vi "Get Step Index from Tree Tag.vi"(11 "Tree Tag":string) -> (2 "Step Param String":string, 3 "Step Index":i32)   [LabVIEW 2024, in "Sequencer with Output Values.lvlib" / "Sequencer with Output Values.lvclass"]
uses:
  Sequencer with Output Values.lvclass
  Global Tree Data.vi
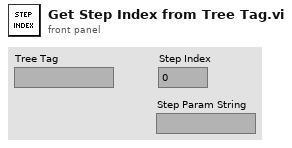
[diagram p1: front panel]
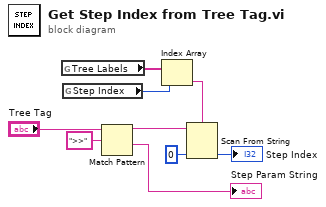
[diagram p0: block diagram]
diagram:
  n1 = global read "Global Tree Data.vi" "Tree Labels"() -> (w5:string[])
  n2 = global read "Global Tree Data.vi" "Step Index"() -> (w2:i32)
  n3 = Match Pattern(string="Tree Tag", regular expression=">>") -> (before substring=w8:string, after substring=→"Step Param String":string)  [unwired: 1 in, 2 out]
  n4 = Index Array(array=w5, index=w2) -> (element=w3:string)
  n5 = Scan From String(format string=w3, input string=w8, default 1=0) -> (output 1=→"Step Index":i32)  [unwired: 2 in, 3 out]
